vi "Look in Cache (element).vi"(9 "element":string, 10 "key":string, 11 "xml cache in":T1) -> (1 "element out":string, 2 "element not found?":bool, 3 "xml cache out":T1)   [LabVIEW 2020, in "Configuration_Helper.lvlib"]
uses:
  Configuration_Helper.lvlib
  _typedefs/xml_1553_cache_type.ctl
  fda7dde8-c448-4cba-b8f0-bccb421290aa.vi
  <vilib>/Comparison/Equal/Equal Functor/Equal Functor.lvclass
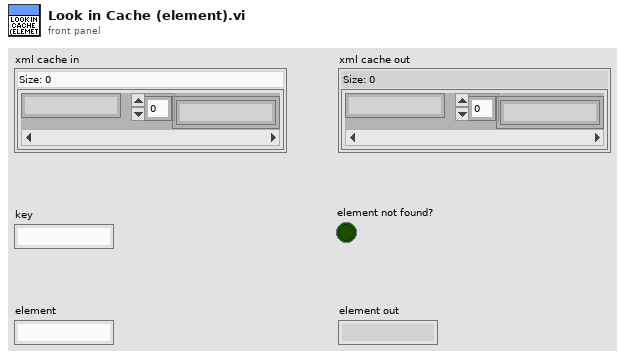
[diagram p1: front panel]
types:
  T1 = typedef "Configuration_Helper.lvlib/xml_1553_cache_type.ctl" = map{string, string[]}
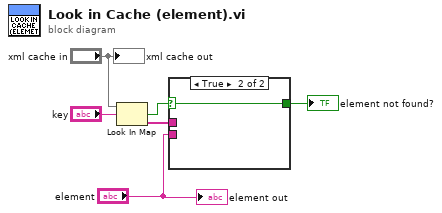
[diagram p0: block diagram]
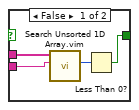
[diagram p2: hidden frame]
diagram:
  n1 = Look In Map(map="xml cache in", key="key") -> (key not found?=w4:bool, value=w3:string[])  [unwired: 1 in]
  n2 = case shown="True" w4 {
    selector: w4 -> [_ w11]
    tunnel: w3 -> [w8 _]
    tunnel: "element" -> [w10 _]
    tunnel: [w9 w11] -> w2
    frame False {
      n3 = call "Search Unsorted 1D Array.vim"("element"=w10, "unsorted 1D array"=w8) -> ("index of element"=w7:i32)  [unwired: 9 in]
      n4 = Less Than 0?(x=w7) -> (x < 0?=w9:bool)
    }
    frame True {
    }
  }
  "element not found?" <- w2
  "xml cache out" <- "xml cache in"
  "element out" <- "element"
